vi "CHECK QUEUE STATUS.vi"(8 "error in (no error)":errorcluster, 11 "StateAuto in":refnum<class "StateAuto.lvclass">) -> (0 "error out":errorcluster, 2 "stateAuto":T1, 3 "StateAuto out":refnum<class "StateAuto.lvclass">)   [LabVIEW 2014, in "LibraryGcode.lvlib" / "StateAuto.lvclass"]
uses:
  StateAuto.lvclass
  StateMachine_Auto.ctl
  StateAuto.lvclass/StateAuto.ctl
panel:
  out "SO QUEUE":i32
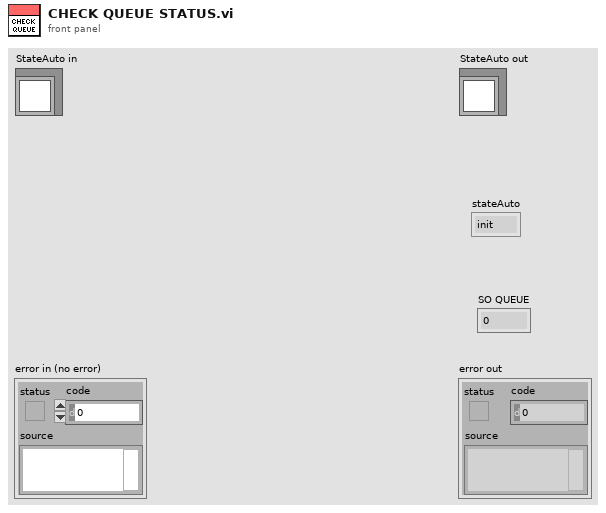
[diagram p1: front panel]
types:
  T1 = typedef "LibraryGcode.lvlib/StateAuto.lvclass/StateMachine_Auto.ctl" = enum16{"init", "checkEMG", "checkStateBoard", "checkQueue", "writeDataQueue", "WaitToRunning", "initNextCommand", "endNextCommand"}
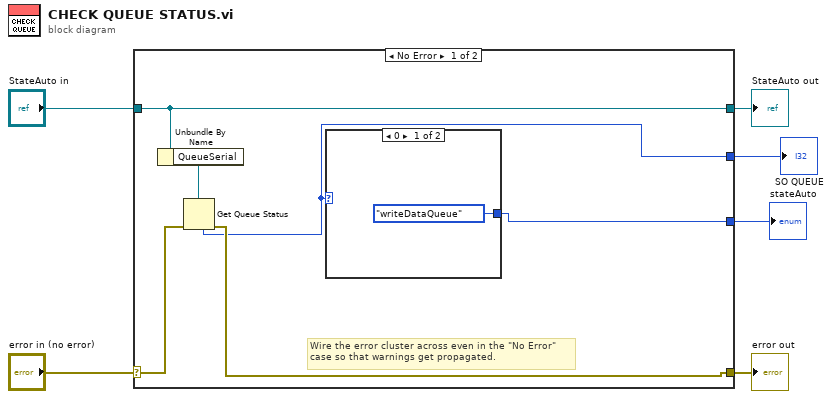
[diagram p0: block diagram]
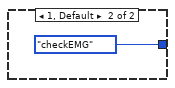
[diagram p2: hidden frame]
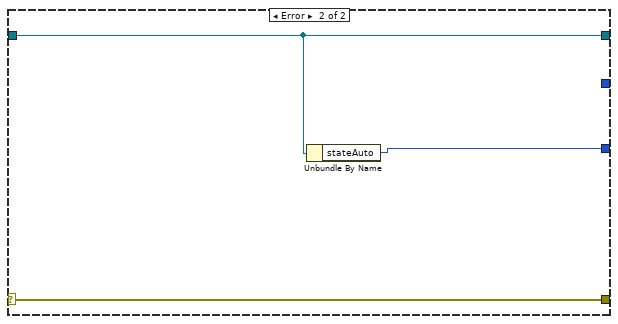
[diagram p3: hidden frame]
diagram:
  n1 = case shown="No Error" "error in (no error)" {
    selector: "error in (no error)" -> [w11 w17]
    tunnel: [w10 w17] -> w5
    tunnel: [w8 w16] -> w3
    tunnel: "StateAuto in" -> [w8 w16]
    tunnel: [w9 w15] -> w2
    tunnel: [w7 _] -> w1
    frame No Error {
      # "Wire the error cluster across even in the \"No Error\"\ncase so that warnings get propagated."
      n2 = Unbundle By Name(w8) -> ("QueueSerial"=w12:refnum<queue>)
      n3 = Get Queue Status(queue=w12, error in (no error)=w11) -> (error out=w10:errorcluster, # elements in queue=w7:i32)  [unwired: 1 in, 6 out]
      n4 = case shown="0" w7 {
        tunnel: [StateMachine_Auto."writeDataQueue" ("stateAuto") StateMachine_Auto."checkEMG" ("stateAuto")] -> w9
        frame 0 {
        }
        frame 1, Default {
        }
      }
    }
    frame Error {
      n5 = Unbundle By Name(w16) -> ("stateAuto"=w15:T1)
    }
  }
  "error out" <- w5
  "StateAuto out" <- w3
  "stateAuto" <- w2
  "SO QUEUE" <- w1
